vi "get_device_info.vi"(0 "device_index (in)":i32, 5 "error in (no error)":errorcluster, 7 "dialog? (T)":bool=TRUE) -> (14 "device_index (out)":i32, 15 "device_info (out)":T1, 19 "error out":errorcluster)   [LabVIEW 2020, in "classes.lvlib" / "_Controller.lvclass"]
uses:
  classes/Controller/_Controller.lvclass
  common/controls/device_info.ctl
  libraries/common.lvlib
  common/controls/models.ctl
  common/controls/device_info_options.ctl
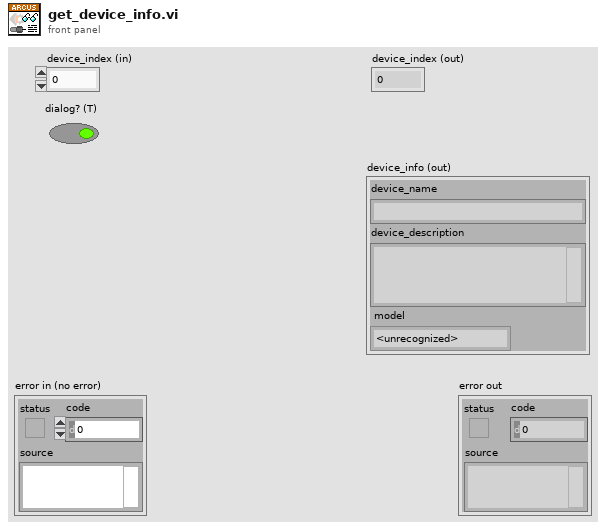
[diagram p1: front panel]
types:
  T1 = typedef "common.lvlib/device_info.ctl" = cluster{"device_name":string, "device_description":string, "model":T2}
  T2 = typedef "common.lvlib/models.ctl" = enum16{"<unrecognized>", "ACE-SDC", "ACE-SDE", "ACE-SXC", "ACE-SXE", "DMX-CAN", "DMX-J-SA", "DMX-K-SA", "DMX-UMD", "PMX-2ED-SA", "PMX-2EX-SA", "PMX-4CX-SA", "PMX-4EX-SA"}
  T3 = typedef "common.lvlib/device_info_options.ctl" = enum16{"device_name", "description"}
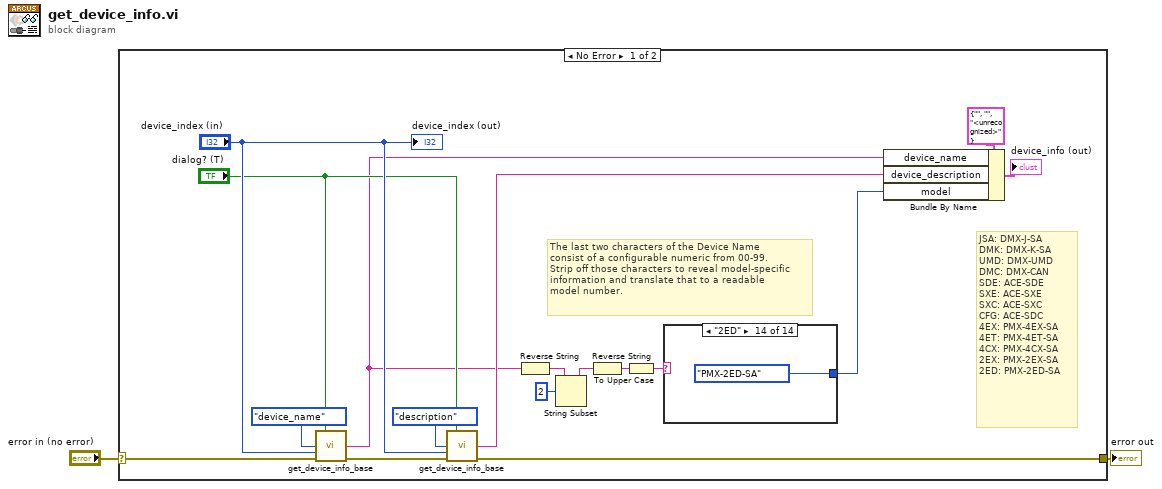
[diagram p0: block diagram]
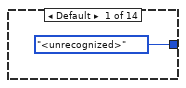
[diagram p2: hidden frame]
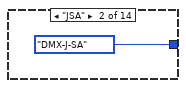
[diagram p3: hidden frame]
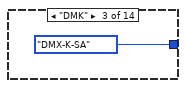
[diagram p4: hidden frame]
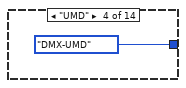
[diagram p5: hidden frame]
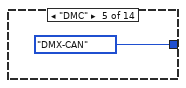
[diagram p6: hidden frame]
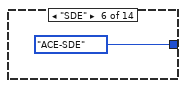
[diagram p7: hidden frame]
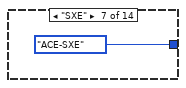
[diagram p8: hidden frame]
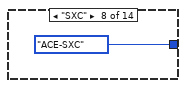
[diagram p9: hidden frame]
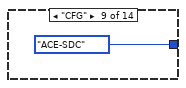
[diagram p10: hidden frame]
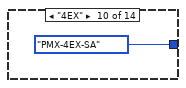
[diagram p11: hidden frame]
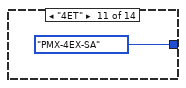
[diagram p12: hidden frame]
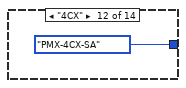
[diagram p13: hidden frame]
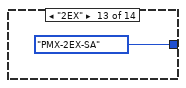
[diagram p14: hidden frame]
diagram:
  n1 = case shown="No Error" "error in (no error)" {
    selector: "error in (no error)" -> [w19 w34]
    tunnel: [w14 w34] -> w1
    frame No Error {
      # "The last two characters of the Device Name\nconsist of a configurable numeric from 00-99.\nStrip off those characters to reveal model-specific\ninformation and translate that to a readable\nmodel number."
      # "JSA: DMX-J-SA\nDMK: DMX-K-SA \nUMD: DMX-UMD\nDMC: DMX-CAN  \nSDE: ACE-SDE\nSXE: ACE-SXE\nSXC: ACE-SXC\nCFG: ACE-SDC \n4EX: PMX-4EX-SA\n4ET: PMX-4ET-SA\n4CX: PMX-4CX-SA\n2EX: PMX-2EX-SA\n2ED: PMX-2ED-SA"
      n2 = call "get_device_info_base.vi"("info_options"=device_info_options."device_name", "device_index"="device_index (in)", "error in (no error)"=w19, "dialog? (T)"="dialog? (T)") -> ("retrieved_info (str)"=w9:string, "error out"=w16:errorcluster)  [unwired: 10 in]
      n3 = call "get_device_info_base.vi"("info_options"=device_info_options."description", "device_index"="device_index (in)", "error in (no error)"=w16, "dialog? (T)"="dialog? (T)") -> ("retrieved_info (str)"=w15:string, "error out"=w14:errorcluster)  [unwired: 10 in]
      n4 = Reverse String(1:w9) -> (0:w8:string)
      n5 = String Subset(string=w8, offset (0)=2) -> (substring=w6:string)  [unwired: 1 in]
      n6 = Reverse String(1:w6) -> (0:w5:string)
      n7 = To Upper Case(1:w5) -> (0:w4:string)
      n8 = case shown="\"2ED\"" w4 {
        tunnel: [models."<unrecognized>" ("model") models."DMX-J-SA" ("model") models."DMX-K-SA" ("model") models."DMX-UMD" ("model") models."DMX-CAN" ("model") models."ACE-SDE" ("model") models."ACE-SXE" ("model") models."ACE-SXC" ("model") models."ACE-SDC" ("model") models."PMX-4EX-SA" ("model") models."PMX-4EX-SA" ("model") models."PMX-4CX-SA" ("model") models."PMX-2EX-SA" ("model") models."PMX-2ED-SA" ("model")] -> w3
        frame Default {
        }
        frame "JSA" {
        }
        frame "DMK" {
        }
        frame "UMD" {
        }
        frame "DMC" {
        }
        frame "SDE" {
        }
        frame "SXE" {
        }
        frame "SXC" {
        }
        frame "CFG" {
        }
        frame "4EX" {
        }
        frame "4ET" {
        }
        frame "4CX" {
        }
        frame "2EX" {
        }
        frame "2ED" {
        }
      }
      n9 = Bundle By Name(cluster=T1 {"device_name"="", "device_description"="", "model"=enum."<unrecognized>"} ("output cluster"), "device_name"=w9, "device_description"=w15, "model"=w3) -> (→"device_info (out)":T1)
      "device_index (out)" <- "device_index (in)"
    }
    frame Error {
    }
  }
  "error out" <- w1
